vi "Get Self Enqueue.vi"(8 "error in (no error)":errorcluster, 11 "Abstruct View in":refnum<class "Abstruct View.lvclass">) -> (0 "error out":errorcluster, 2 "Self Enqueuer":refnum<class "Message Enqueuer.lvclass">, 3 "Abstruct View out":refnum<class "Abstruct View.lvclass">)   [LabVIEW 2020, in "Abstruct View.lvlib" / "Abstruct View.lvclass"]
uses:
  Abstruct View.lvclass
  C:/Program Files (x86)/National Instruments/LabVIEW 2020/vi.lib/ActorFramework/Actor/Actor.lvclass
  <vilib>/ActorFramework/Message Enqueuer/Message Enqueuer.lvclass
  <vilib>/ActorFramework/Actor/Actor.lvclass/Actor.ctl
  <vilib>/ActorFramework/Message Enqueuer/Message Enqueuer.lvclass/Message Enqueuer.ctl
  <vilib>/ActorFramework/Message Enqueuer/Init from Existing Queue.vi
  Abstruct View.lvclass/Abstruct View.ctl
  <vilib>/ActorFramework/Actor/Actor.lvclass
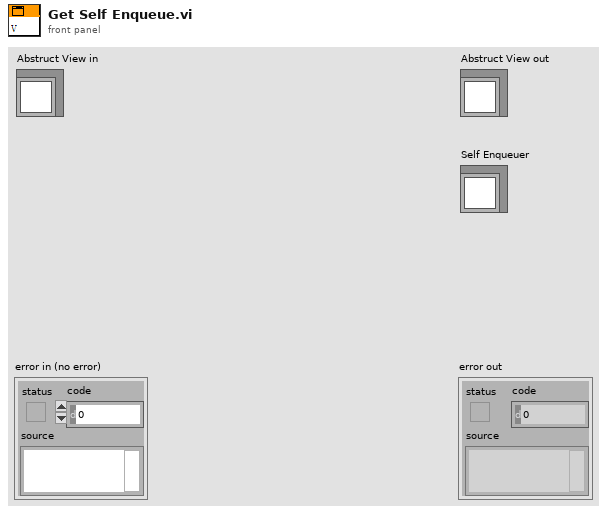
[diagram p1: front panel]
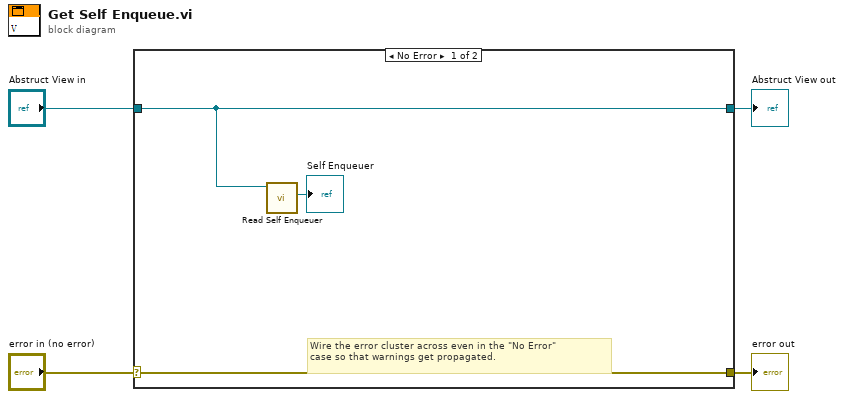
[diagram p0: block diagram]
diagram:
  n1 = case shown="No Error" "error in (no error)" {
    selector: "error in (no error)" -> [w7 w9]
    tunnel: [w7 w9] -> w3
    tunnel: [w6 w8] -> w1
    tunnel: "Abstruct View in" -> [w6 w8]
    frame No Error {
      # "Wire the error cluster across even in the \"No Error\"\ncase so that warnings get propagated."
      n2 = call <vilib>:"Read Self Enqueuer.vi"("Actor"=w6) -> ("Self Enqueuer"=→"Self Enqueuer":refnum<class "Message Enqueuer.lvclass">)  [unwired: 10 in]
    }
    frame Error {
    }
  }
  "error out" <- w3
  "Abstruct View out" <- w1
